vi "File check 1.0.vi"(8 "error in (no error)":errorcluster, 9 "Bool Refnum":refnum<vi>, 10 "reference":refnum<vi>, 11 "path":path) -> (0 "error out":errorcluster, 3 "Next State":string)   [LabVIEW 2016]
uses:
  Type Defs/File Check 2.0 control.ctl
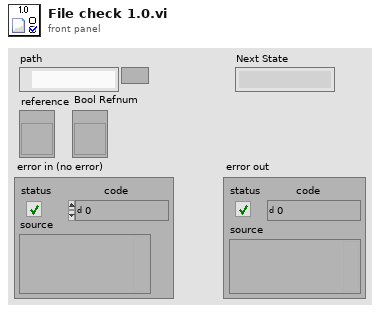
[diagram p1: front panel]
types:
  T1 = typedef "File Check 2.0 control.ctl" = enum16{"File Check", "Secondary check", "Refresh Google Drive"}
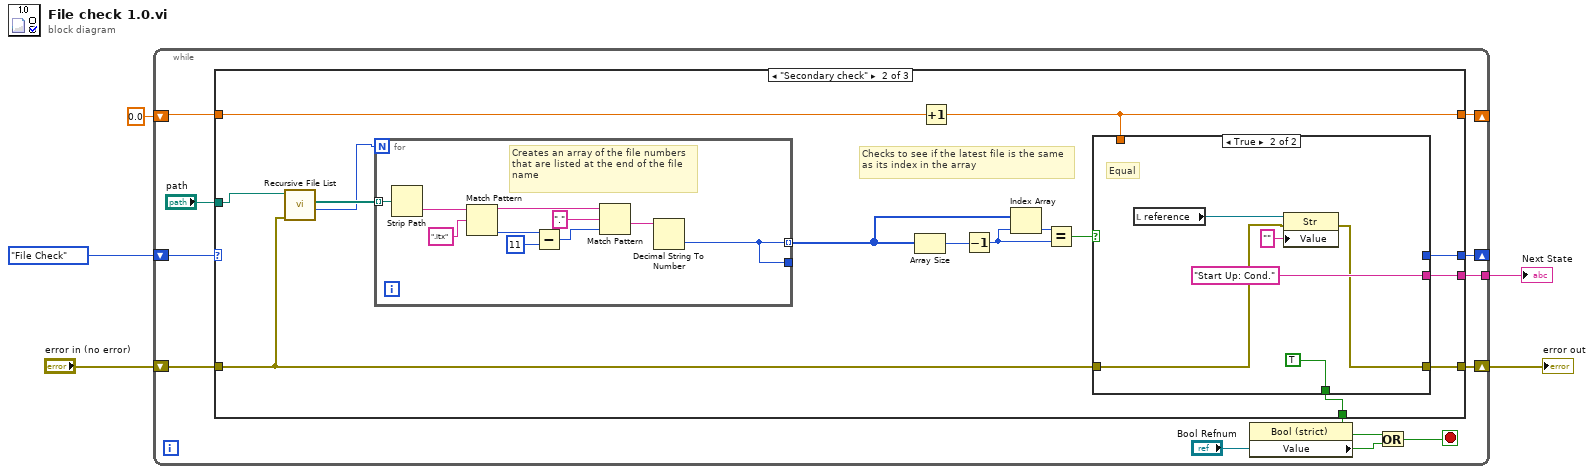
[diagram p0: block diagram]
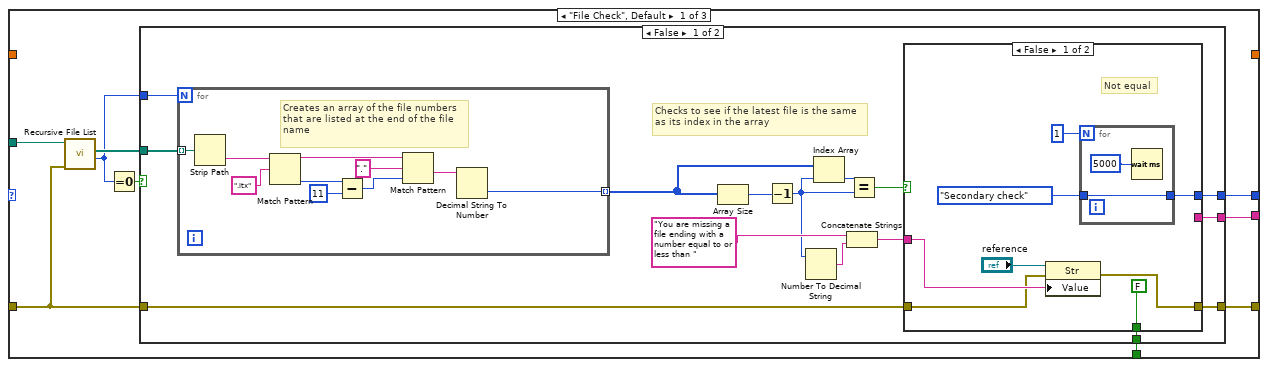
[diagram p2: hidden frame]
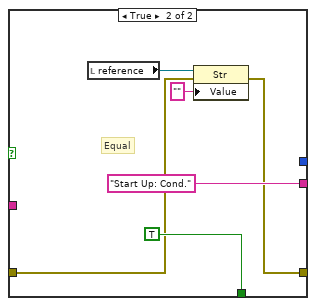
[diagram p3: hidden frame]
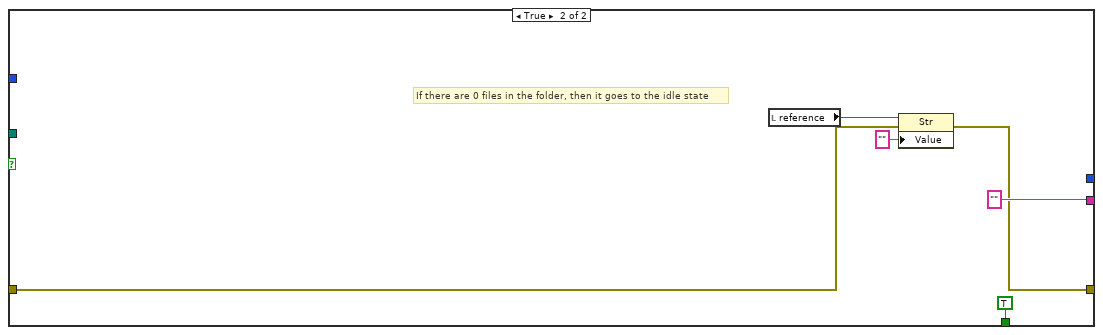
[diagram p4: hidden frame]
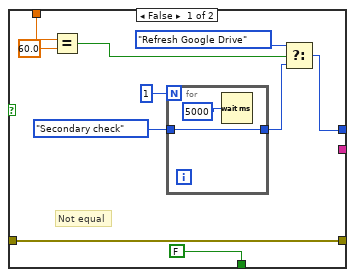
[diagram p5: hidden frame]
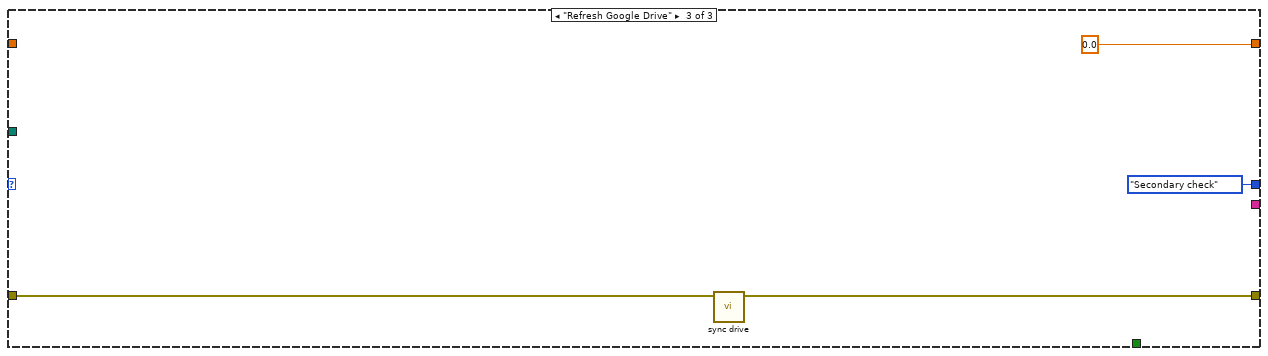
[diagram p6: hidden frame]
diagram:
  n1 = while {
    tunnel: [w17] -> w5
    shift-right: [w15] -> _
    shift-left: File_Check_2.0_control."File Check" -> [w14]
    shift-right: [w13] -> w3
    shift-left: "error in (no error)" -> [w12]
    shift-right: [w10] -> _
    shift-left: 0.0 -> [w11]
    stop <- w8 stop-if-true
    n2 = case shown="\"Secondary check\"" w14 {
      tunnel: [w25 w83 _] -> w17
      tunnel: [w23 w82 _] -> w9
      tunnel: "path" -> [w20 w79 _]
      tunnel: [w24 w77 File_Check_2.0_control."Secondary check"] -> w15
      tunnel: w12 -> [w19 w74 w118]
      tunnel: [w18 w78 w119] -> w13
      tunnel: w11 -> [_ w76 _]
      tunnel: [_ w75 0.0] -> w10
      frame "File Check", Default {
        n3 = call <vilib>:"Recursive File List.vi"("error in (no error)"=w19, "Folder Path"=w20) -> ("Number of Files"=w22:i32, "All Files in Dir"=w26:path[])  [unwired: 6 in, 2 out]
        n4 = Equal To 0?(x=w22) -> (x = 0?=w21:bool)
        n5 = case shown="False" w21 {
          tunnel: w26 -> [w41 _]
          tunnel: [w36 "" ("Message")] -> w25
          tunnel: [w35 _] -> w24
          tunnel: [w34 TRUE] -> w23
          tunnel: w22 -> [w33 _]
          tunnel: w19 -> [w28 w69]
          tunnel: [w27 w68] -> w18
          frame False {
            # "Checks to see if the latest file is the same as its index in the array"
            n6 = for {
              N: w33 -> [_]
              tunnel: [w58] -> w37 mode=indexing
              tunnel: w41 -> [w59] mode=indexing
              # "Creates an array of the file numbers that are listed at the end of the file name"
              n7 = Strip Path(path=w59) -> (name=w67:string)  [unwired: 1 out]
              n8 = Match Pattern(string=w67, regular expression=".itx") -> (before substring=w62:string, offset past match=w65:i32)  [unwired: 1 in, 2 out]
              n9 = Subtract(x=w65, y=11) -> (x-y=w63:i32)
              n10 = Match Pattern(string=w62, regular expression=".", offset (0)=w63) -> (after substring=w60:string)  [unwired: 3 out]
              n11 = Decimal String To Number(string=w60) -> (number=w58:i32)  [unwired: 2 in, 1 out]
            }
            n12 = Array Size(array=w37) -> (size(s)=w40:i32)
            n13 = Decrement(x=w40) -> (x-1=w30:i32)
            n14 = Number To Decimal String(number=w30) -> (decimal integer string=w31:string)  [unwired: 1 in]
            n15 = Index Array(array=w37, index=w30) -> (element=w39:i32)
            n16 = Concatenate Strings("You are missing a file ending with a number equal to or less than ", w31) -> (w29:string)
            n17 = Equal?(x=w39, y=w30) -> (x = y?=w38:bool)
            n18 = case shown="False" w38 {
              tunnel: [_ "Start Up: Cond." ("Message")] -> w36
              tunnel: [FALSE TRUE] -> w34
              tunnel: [w49 _] -> w35
              tunnel: w29 -> [w44 _]
              tunnel: w28 -> [w43 w53]
              tunnel: [w42 w52] -> w27
              frame False {
                # "Not equal"
                n19 = property class="Str"(reference="reference", error in=w43, "Value"=w44) -> (error out=w42:errorcluster)  [unwired: 1 out]
                n20 = for {
                  N: 1 -> [_]
                  tunnel: [w50] -> w49
                  tunnel: File_Check_2.0_control."Secondary check" -> [w50]
                  n21 = Wait (ms)(milliseconds to wait=u32 5000) -> ()  [unwired: 1 out]
                }
              }
              frame True {
                # "Equal"
                n22 = local read "reference"() -> (w55:refnum<vi>)
                n23 = property class="Str"(reference=w55, error in=w53, "Value"="") -> (error out=w52:errorcluster)  [unwired: 1 out]
              }
            }
          }
          frame True {
            # "If there are 0 files in the folder, then it goes to the idle state"
            n24 = local read "reference"() -> (w71:refnum<vi>)
            n25 = property class="Str"(reference=w71, error in=w69, "Value"="") -> (error out=w68:errorcluster)  [unwired: 1 out]
          }
        }
      }
      frame "Secondary check" {
        # "Checks to see if the latest file is the same as its index in the array"
        n26 = call <vilib>:"Recursive File List.vi"("error in (no error)"=w74, "Folder Path"=w79) -> ("Number of Files"=w81:i32, "All Files in Dir"=w88:path[])  [unwired: 6 in, 2 out]
        n27 = for {
          N: w81 -> [_]
          tunnel: [w107] -> w84 mode=indexing
          tunnel: w88 -> [w108] mode=indexing
          tunnel: [w107] -> _
          # "Creates an array of the file numbers that are listed at the end of the file name"
          n28 = Strip Path(path=w108) -> (name=w116:string)  [unwired: 1 out]
          n29 = Match Pattern(string=w116, regular expression=".itx") -> (before substring=w111:string, offset past match=w114:i32)  [unwired: 1 in, 2 out]
          n30 = Subtract(x=w114, y=11) -> (x-y=w112:i32)
          n31 = Match Pattern(string=w111, regular expression=".", offset (0)=w112) -> (after substring=w109:string)  [unwired: 3 out]
          n32 = Decimal String To Number(string=w109) -> (number=w107:i32)  [unwired: 2 in, 1 out]
        }
        n33 = Array Size(array=w84) -> (size(s)=w87:i32)
        n34 = Increment(x=w76) -> (x+1=w75:dbl)
        n35 = Decrement(x=w87) -> (x-1=w80:i32)
        n36 = Index Array(array=w84, index=w80) -> (element=w86:i32)
        n37 = Equal?(x=w86, y=w80) -> (x = y?=w85:bool)
        n38 = case shown="True" w85 {
          tunnel: [_ "Start Up: Cond." ("Message")] -> w83
          tunnel: [FALSE TRUE] -> w82
          tunnel: w74 -> [w95 w102]
          tunnel: [w95 w101] -> w78
          tunnel: [w90 _] -> w77
          tunnel: w75 -> [w94 _]
          frame False {
            # "Not equal"
            n39 = Equal?(x=w94, y=60.0) -> (x = y?=w89:bool)
            n40 = for {
              N: 1 -> [_]
              tunnel: File_Check_2.0_control."Secondary check" -> [w99]
              tunnel: [w99] -> w91
              n41 = Wait (ms)(milliseconds to wait=u32 5000) -> ()  [unwired: 1 out]
            }
            n42 = Select(t=File_Check_2.0_control."Refresh Google Drive", s=w89, f=w91) -> (s? t:f=w90:T1)
          }
          frame True {
            # "Equal"
            n43 = local read "reference"() -> (w104:refnum<vi>)
            n44 = property class="Str"(reference=w104, error in=w102, "Value"="") -> (error out=w101:errorcluster)  [unwired: 1 out]
          }
        }
      }
      frame "Refresh Google Drive" {
        n45 = call "sync drive.vi"("error in (no error)"=w118) -> ("error out"=w119:errorcluster)  [unwired: 10 in]
      }
    }
    n46 = property class="Bool (strict)"(reference="Bool Refnum") -> ("Value"=w6:bool)  [unwired: 1 in, 2 out]
    n47 = Or(x=w9, y=w6) -> (x .or. y?=w8:bool)
  }
  "Next State" <- w5
  "error out" <- w3
